vi "TAV.vi"(0 "System no.":i32=1 min=1 max=4 step=1, 1 "Board":i32=1 min=1 max=5 step=1, 2 "Set":u16(ring) items=["Value", "Range", "Power unit"], 3 "Analog value":dbl format="%.6f", 5 "error in":errorcluster, 6 "Range":dbl=0.1, 7 "Power unit":u16(ring) items=["µW", "mW", "dBm"]) -> (14 "Controller error":bool, 19 "error out":errorcluster)   [LabVIEW 2026]
doc: "Sets range and power unit for optical head.\n\nC-887, F-206, M-8X0: Only for GCS syntax version = GCS 1.0 (check with CSV?.vi. If CSV?.vi is not supported, syntax version is GCS 1.0)."
panel:
  # "Sets range and power unit for optical head."
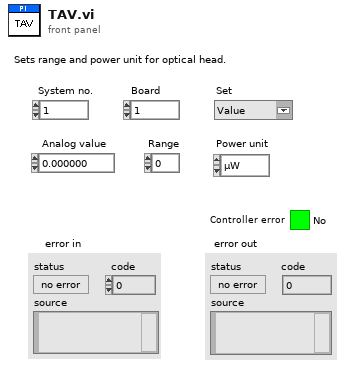
[diagram p1: front panel]
types:
  T1 = enum16{"Disable error check", "Force error check", "Use global settings"}
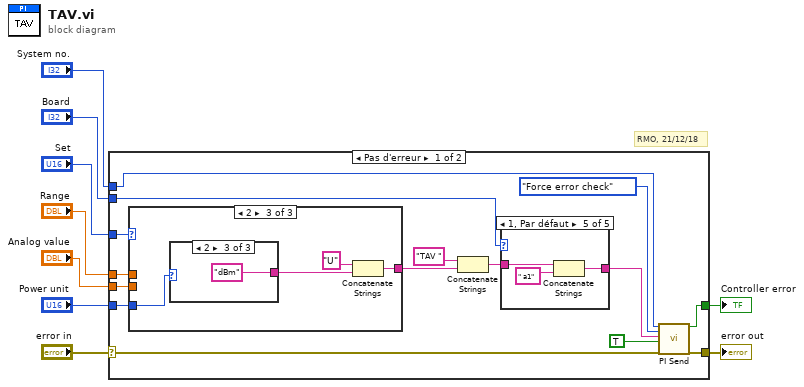
[diagram p0: block diagram]
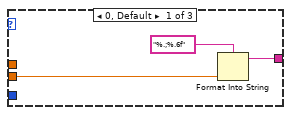
[diagram p2: hidden frame]
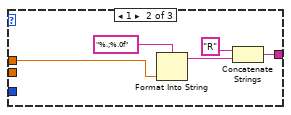
[diagram p3: hidden frame]
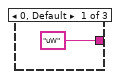
[diagram p4: hidden frame]
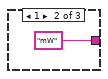
[diagram p5: hidden frame]
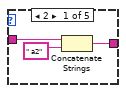
[diagram p6: hidden frame]
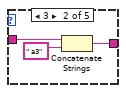
[diagram p7: hidden frame]
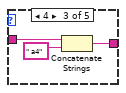
[diagram p8: hidden frame]
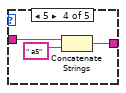
[diagram p9: hidden frame]
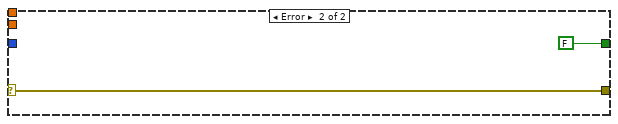
[diagram p10: hidden frame]
diagram:
  # "RMO, 21/12/18"
  n1 = case shown="Pas d'erreur" "error in" {
    selector: "error in" -> [w13 w55]
    tunnel: "System no." -> [w18 _]
    tunnel: [w11 w55] -> w8
    tunnel: [w10 FALSE] -> w5
    tunnel: "Board" -> [w24 _]
    tunnel: "Range" -> [w23 _]
    tunnel: "Power unit" -> [w17 _]
    tunnel: "Set" -> [w16 _]
    tunnel: "Analog value" -> [w15 _]
    frame No Error {
      n2 = case shown="2" w16 {
        tunnel: w23 -> [_ w32 _]
        tunnel: [w26 w28 w33] -> w14
        tunnel: w17 -> [_ _ w36]
        tunnel: w15 -> [w25 _ _]
        frame 0, Default {
          n3 = Format Into String(format string="%.;%.6f" ("Format String"), w25) -> (resulting string=w26:string)  [unwired: 2 in, 1 out]
        }
        frame 1 {
          n4 = Format Into String(format string="%.;%.0f" ("Format String"), w32) -> (resulting string=w29:string)  [unwired: 2 in, 1 out]
          n5 = Concatenate Strings("R", w29) -> (w28:string)
        }
        frame 2 {
          n6 = case shown="2" w36 {
            tunnel: ["uW" "mW" "dBm"] -> w34
            frame 0, Default {
            }
            frame 1 {
            }
            frame 2 {
            }
          }
          n7 = Concatenate Strings("U", w34) -> (w33:string)
        }
      }
      n8 = Concatenate Strings("TAV ", w14) -> (w21:string)
      n9 = case shown="1, Par défaut" w24 {
        tunnel: w21 -> [w42 w45 w48 w51 w54]
        tunnel: [w40 w43 w46 w49 w52] -> w20
        frame 2 {
          n10 = Concatenate Strings(w42, " a2" ("Substring")) -> (w40:string)
        }
        frame 3 {
          n11 = Concatenate Strings(w45, " a3" ("Substring")) -> (w43:string)
        }
        frame 4 {
          n12 = Concatenate Strings(w48, " a4" ("Substring")) -> (w46:string)
        }
        frame 5 {
          n13 = Concatenate Strings(w51, " a5" ("Substring")) -> (w49:string)
        }
        frame 1, Default {
          n14 = Concatenate Strings(w54, " a1" ("Substring")) -> (w52:string)
        }
      }
      n15 = call "PI Send.vi"("System no."=w18, "Error check settings"=T1."Force error check", "String to send"=w20, "Attach termination char.?"=TRUE ("Attach Linefeed?"), "error in"=w13) -> ("Controller error"=w10:bool, "error out"=w11:errorcluster)  [unwired: 1 in, 12 out]
    }
    frame Error {
    }
  }
  "error out" <- w8
  "Controller error" <- w5
